vi "headers_April2018.vi"(10 "Sample names":T1={"QCM1 sample name"="aQCM2", "QCM2 sample name"="aQCM2", "QCM3 sample name"="aQCM3", "QCM4 sample name"="aQCM4", "QCM5 sample name"="aQCM5", "QCM6 sample name"="aQCM6", "SRS sample name"="sample_SRS", "Keithley 2420 sample name"="Keithley2420", "Keithley 6430 sample name"="Keithley6430", "Keithley 2100 sample name"="Keithley6430", "Gas"="aQCM2", "Vapor"="aQCM2", "Experiment Notes"=""}) -> (2 "data headers":string[](array[string]))   [LabVIEW 2014]
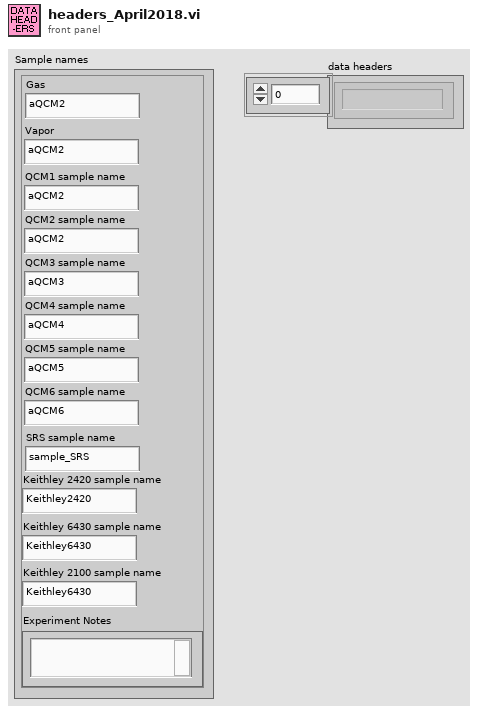
[diagram p1: front panel]
types:
  T1 = cluster{"QCM1 sample name":string, "QCM2 sample name":string, "QCM3 sample name":string, "QCM4 sample name":string, "QCM5 sample name":string, "QCM6 sample name":string, "SRS sample name":string, "Keithley 2420 sample name":string, "Keithley 6430 sample name":string, "Keithley 2100 sample name":string, "Gas":string, "Vapor":string, "Experiment Notes":string}
  T2 = cluster{string, string, string, string, string, string}
  T3 = cluster{"element":string, "element":string, "element":string, "element":string}
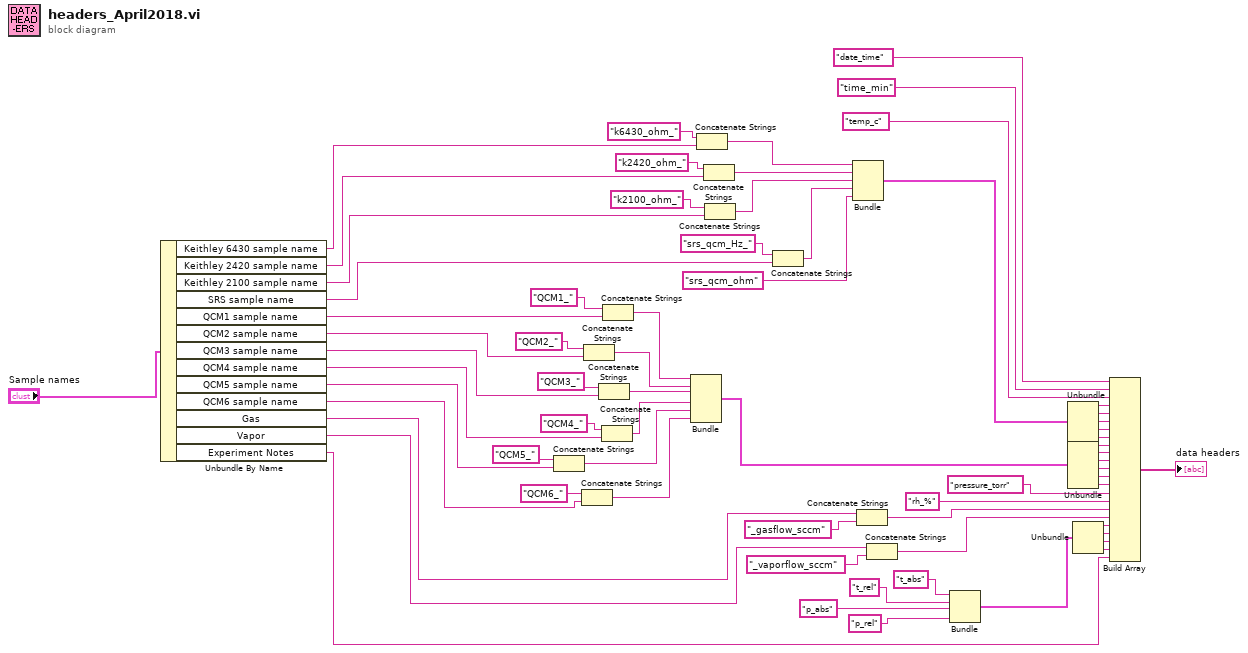
[diagram p0: block diagram]
diagram:
  n1 = Unbundle By Name("Sample names") -> ("Keithley 6430 sample name"=w27:string, "Keithley 2420 sample name"=w26:string, "Keithley 2100 sample name"=w25:string, "SRS sample name"=w24:string, "QCM1 sample name"=w61:string, "QCM2 sample name"=w58:string, "QCM3 sample name"=w56:string, "QCM4 sample name"=w54:string, "QCM5 sample name"=w51:string, "QCM6 sample name"=w50:string, "Gas"=w38:string, "Vapor"=w37:string, "Experiment Notes"=w29:string)
  n2 = Concatenate Strings("QCM5_" ("string"), w51) -> (w32:string)
  n3 = Concatenate Strings("QCM6_" ("string"), w50) -> (w31:string)
  n4 = Concatenate Strings("QCM2_" ("string"), w58) -> (w35:string)
  n5 = Concatenate Strings("QCM3_" ("string"), w56) -> (w34:string)
  n6 = Concatenate Strings("QCM4_" ("string"), w54) -> (w33:string)
  n7 = Concatenate Strings("QCM1_" ("string"), w61) -> (w36:string)
  n8 = Bundle(w36, w35, w34, w33, w32, w31) -> (w30:T2)  [unwired: 1 in]
  n9 = Concatenate Strings("k6430_ohm_", w27) -> (w47:string)
  n10 = Concatenate Strings("k2420_ohm_" ("element"), w26) -> (w46:string)
  n11 = Concatenate Strings("k2100_ohm_" ("element"), w25) -> (w45:string)
  n12 = Concatenate Strings("srs_qcm_Hz_", w24) -> (w13:string)
  n13 = Bundle(w47, w46, w45, w13, "srs_qcm_ohm") -> (w44:cluster{string, string, string, string, string})  [unwired: 1 in]
  n14 = Concatenate Strings(w38, "_gasflow_sccm" ("element")) -> (w15:string)
  n15 = Concatenate Strings(w37, "_vaporflow_sccm" ("element")) -> (w14:string)
  n16 = Bundle("element"="t_abs", "element"="t_rel", "element"="p_abs", "element"="p_rel") -> (w5:T3)  [unwired: 1 in]
  n17 = Unbundle(w44) -> (w43:string, w42:string, w41:string, w11:string, w10:string)
  n18 = Unbundle(w30) -> (w23:string, w22:string, w21:string, w20:string, w19:string, w18:string)
  n19 = Unbundle(w5) -> ("element"=w4:string, "element"=w3:string, "element"=w2:string, "element"=w1:string)
  n20 = Build Array("date_time", "time_min", "temp_c", w43, w42, w41, w11, w10, w23, w22, w21, w20, w19, w18, "pressure_torr" ("element"), "rh_%" ("element"), w15, w14, w4, w3, w2, w1, w29) -> (→"data headers":string[])
